vi "Runtime Conditional Disable Structure.vi"   [LabVIEW 2017]
doc: "Use this VI as a template. This VI is a default VI that executes when the run time engine is on."
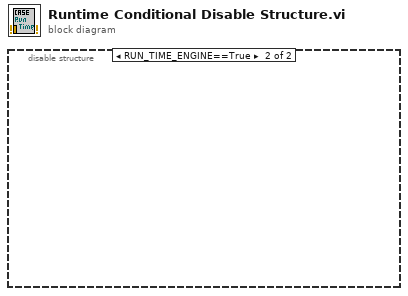
[diagram p0: block diagram]
diagram:
  n1 = disable-structure shown="RUN_TIME_ENGINE==True" {
    frame condition #0 (active) {
    }
    frame condition #1 {
    }
  }
